vi "自动添加所有参数数据.vi"() -> ()   [LabVIEW 2016, in "数据查询.lvlib"]
uses:
  <vilib>/Utility/sysdir.llb/System Directory Type.ctl
  <vilib>/addons/database/Connection.llb/DB Tools Open Connec (String).vi
  <vilib>/Utility/config.llb/Read Key (String).vi
  <vilib>/Utility/config.llb/Write Key (String).vi
  <vilib>/addons/database/NI_Database_API.lvlib
  <vilib>/Utility/config.llb/NI_LVConfig.lvlib
panel:
  in  "error in (no error)":errorcluster
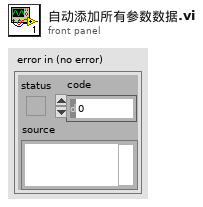
[diagram p1: front panel]
types:
  T1 = typedef "System Directory Type.ctl" = i32
  T2 = typedef "NI_Database_API.lvlib/Conn ObjectReference.ctl" = refnum<k1>
  T3 = typedef "NI_LVConfig.lvlib/Config Data RefNum.ctl" = refnum<k1>
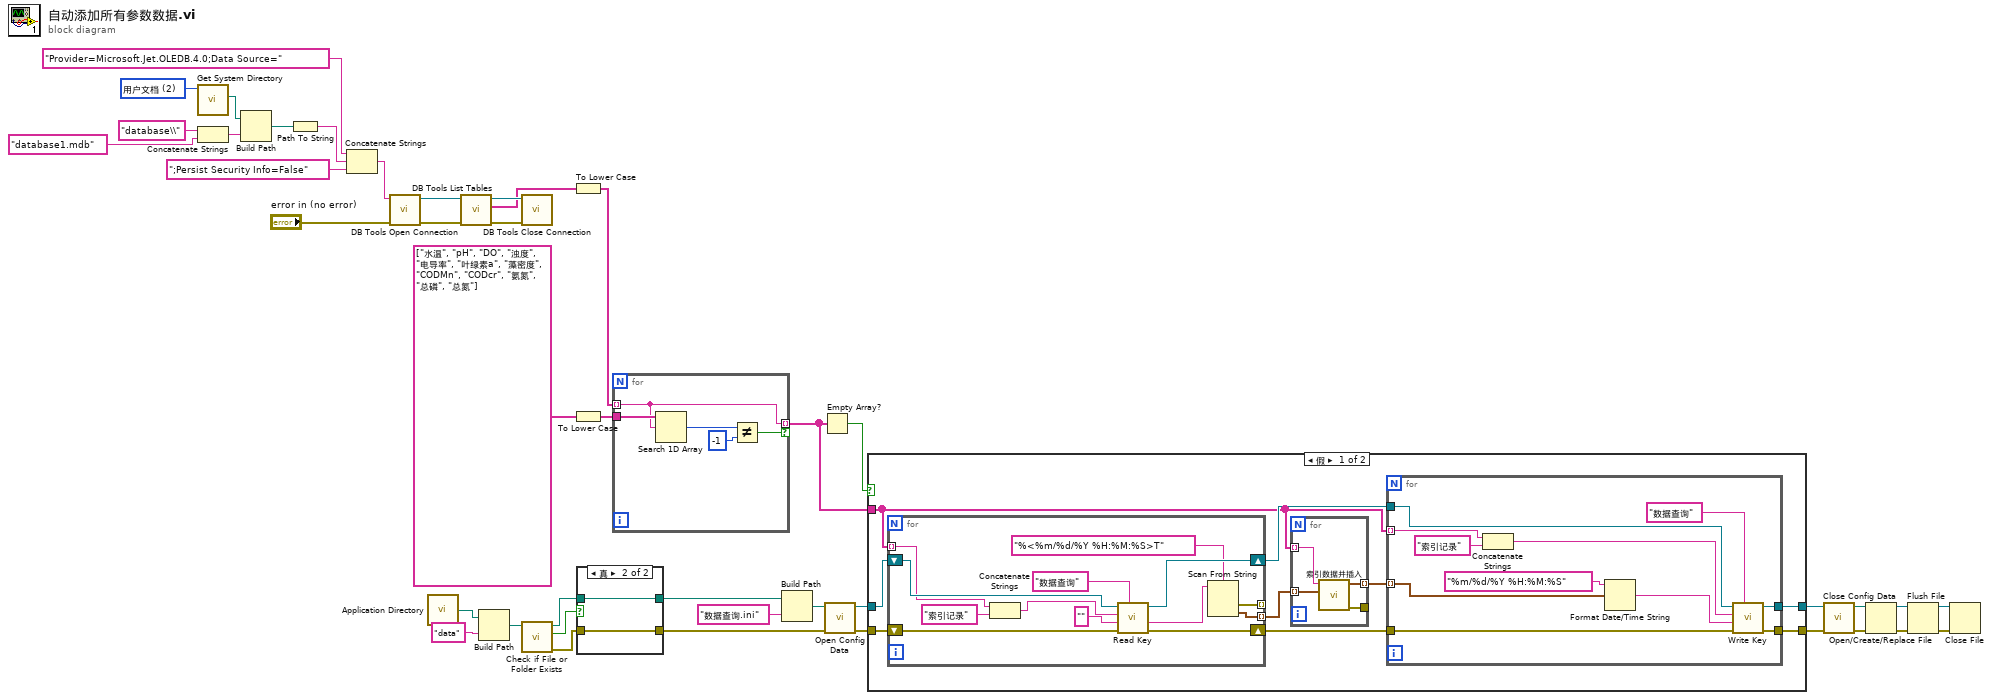
[diagram p0: block diagram]
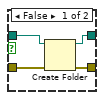
[diagram p3: hidden frame]
diagram:
  w41 = T1 2 items=["用户目录"=0, "用户桌面"=1, "用户文档"=2, "用户应用程序数据"=3, "用户设置"=4, "用户临时目录"=5, "公共文档"=6, "公共应用程序数据"=7, "公共设置"=8, "公共缓存"=13, "系统核心库"=9, "系统安装库"=10, "应用程序文件"=11, "启动盘根目录"=12] ("system directory type")
  n1 = call <vilib>:"Get System Directory.vi"("system directory type"=w41) -> ("system directory"=w39:path)  [unwired: 10 in]
  n2 = Concatenate Strings("database\\" ("condition"), "database1.mdb" ("字符串")) -> (w33:string)
  n3 = Build Path(base path=w39, name or relative path=w33) -> (appended path=w38:path)
  n4 = Path To String(path=w38) -> (string=w37:string)
  n5 = Concatenate Strings("Provider=Microsoft.Jet.OLEDB.4.0;Data Source=" ("condition"), w37, ";Persist Security Info=False" ("condition")) -> (w35:string)
  n6 = call-poly <vilib>:"DB Tools Open Connection.vi"("error in (no error)"="error in (no error)", "connection information"=w35) -> ("error out"=w29:errorcluster, "connection reference"=w30:T2)  [unwired: 6 in]
  n7 = call <vilib>:"Application Directory.vi"() -> ("Application Directory"=w15:path)
  n8 = call <vilib>:"DB Tools List Tables.vi"("error in (no error)"=w29, "connection reference"=w30) -> ("error out"=w28:errorcluster, "tables"=w24:string[], "connection reference out"=w27:T2)  [unwired: 3 in]
  n9 = Build Path(base path=w15, name or relative path="data" ("名称或相对路径")) -> (appended path=w17:path)
  n10 = call <vilib>:"DB Tools Close Connection.vi"("error in (no error)"=w28, "connection reference"=w27) -> ()  [unwired: 5 in, 1 out]
  n11 = call <vilib>:"Check if File or Folder Exists.vi"("path"=w17) -> ("error out"=w20:errorcluster, "file or folder exists?"=w18:bool, "dup path"=w19:path)  [unwired: 8 in]
  n12 = To Lower Case(string=w24) -> (all lower case string=w23:string[])
  n13 = To Lower Case(string=string[] ["水温", "pH", "DO", "浊度", "电导率", "叶绿素a", "藻密度", "CODMn", "CODcr", "氨氮", "总磷", "总氮"]) -> (all lower case string=w25:string[])
  n14 = case shown="真" w18 {
    tunnel: w19 -> [w45 w47]
    tunnel: w20 -> [w44 w46]
    tunnel: [w43 w47] -> w21
    tunnel: [w42 w46] -> w6
    frame False {
      n15 = Create Folder(path (use dialog)=w45, error in=w44) -> (created path=w43:path, error out=w42:errorcluster)  [unwired: 1 in, 1 out]
    }
    frame True {
    }
  }
  n16 = for {
    tunnel: w23 -> [w49] mode=indexing
    tunnel: w25 -> [w52]
    tunnel: [w49] -> w3 mode=indexing if=w48
    n17 = Search 1D Array(1D array=w52, element=w49) -> (index of element=w51:i32)  [unwired: 1 in]
    n18 = Not Equal?(x=w51, y=-1) -> (x != y?=w48:bool)
  }
  n19 = Build Path(base path=w21, name or relative path="数据查询.ini" ("名称或相对路径")) -> (appended path=w14:path)
  n20 = Empty Array?(array=w3) -> (empty?=w2:bool)
  n21 = call <vilib>:"Open Config Data.vi"("error in (no error)"=w6, "configuration file path"=w14) -> ("error out"=w4:errorcluster, "refnum"=w5:T3)  [unwired: 7 in, 1 out]
  n22 = case shown="假" w2 {
    tunnel: [w60 w91] -> w8
    tunnel: [w59 w90] -> w7
    tunnel: w5 -> [w58 w91]
    tunnel: w4 -> [w57 w90]
    tunnel: w3 -> [w54 _]
    frame False {
      n23 = for {
        shift-right: [w83] -> w56
        shift-left: w58 -> [w85]
        shift-right: [w82] -> w55
        shift-left: w57 -> [w84]
        tunnel: w54 -> [w78] mode=indexing
        tunnel: [w74] -> w53 mode=indexing
        tunnel: [w73] -> _ mode=indexing
        n24 = Concatenate Strings(w78, "索引记录" ("key")) -> (w79:string)
        n25 = call-poly <vilib>:"Read Key.vi"("section"="数据查询", "error in (no error)"=w84, "default value"="", "key"=w79, "refnum"=w85) -> ("error out"=w82:errorcluster, "value"=w76:string, "refnum out"=w83:T3)  [unwired: 3 in, 1 out]
        n26 = Scan From String(format string="%<%m/%d/%Y %H:%M:%S>T" ("格式字符串"), input string=w76) -> (error out=w73:errorcluster, output 1=w74:timestamp)  [unwired: 3 in, 2 out]
      }
      n27 = for {
        tunnel: w53 -> [w89] mode=indexing
        tunnel: w54 -> [w88] mode=indexing
        tunnel: [w87] -> _
        tunnel: [w86] -> w61 mode=indexing
        n28 = call "索引数据并插入.vi"("索引记录"=w89, "table"=w88) -> ("error out"=w87:errorcluster, "最新索引记录"=w86:timestamp)  [unwired: 8 in]
      }
      n29 = for {
        tunnel: w54 -> [w71] mode=indexing
        tunnel: w61 -> [w68] mode=indexing
        tunnel: w56 -> [w66]
        tunnel: w55 -> [w65]
        tunnel: [w64] -> w60
        tunnel: [w63] -> w59
        n30 = Concatenate Strings(w71, "索引记录" ("key")) -> (w69:string)
        n31 = Format Date/Time String(time format string (%c)="%m/%d/%Y %H:%M:%S" ("时间格式字符串(%c)"), seconds (now)=w68) -> (date/time string=w67:string)  [unwired: 1 in]
        n32 = call-poly <vilib>:"Write Key.vi"("section"="数据查询", "error in (no error)"=w65, "value"=w67, "key"=w69, "refnum"=w66) -> ("error out"=w63:errorcluster, "refnum out"=w64:T3)  [unwired: 4 in, 1 out]
      }
    }
    frame True {
    }
  }
  n33 = call <vilib>:"Close Config Data.vi"("error in (no error)"=w7, "refnum"=w8) -> ("error out"=w13:errorcluster, "file path"=w1:path)  [unwired: 8 in]
  n34 = Open/Create/Replace File(file path (use dialog)=w1, error in=w13) -> (refnum out=w9:refnum<file>, error out=w10:errorcluster)  [unwired: 4 in, 1 out]
  n35 = Flush File(refnum=w9, error in=w10) -> (refnum out=w11:refnum<file>, error out=w12:errorcluster)
  n36 = Close File(refnum=w11, error in=w12) -> ()  [unwired: 2 out]
